vi "Default Position.vi"(0 "Selected Doc[]":refnum<class "Document.lvclass">[](array[class]), 5 "Position[]":T1[](array[typedef]), 11 "error in":errorcluster) -> (4 "Selected Doc[]":refnum<class "Document.lvclass">[](array[class]), 6 "Position[]":T1[](array[typedef]), 15 "error Out":errorcluster)   [LabVIEW 2016, in "LV MDI.lvclass"]
doc: "Set Default position for window."
uses:
  LV MDI.lvclass
  protected/Postion.ctl
  Document/Document base/Document.lvclass
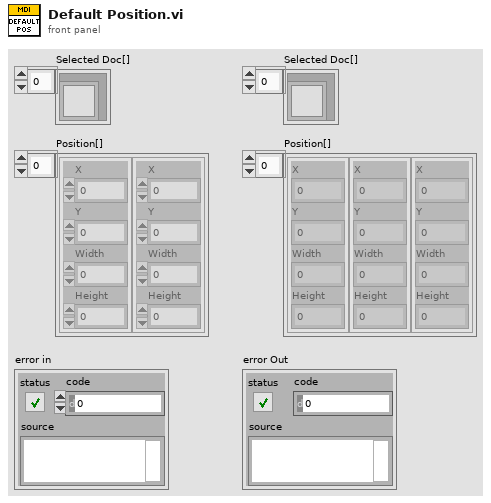
[diagram p1: front panel]
types:
  T1 = typedef "Postion.ctl" = cluster{"X":i32, "Y":i32, "Width":i32, "Height":i32}
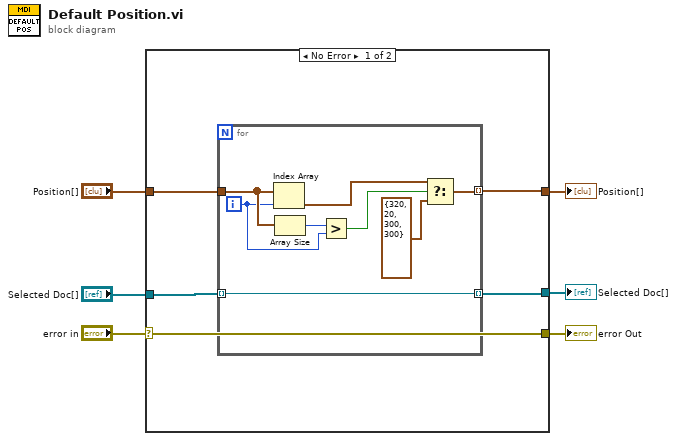
[diagram p0: block diagram]
diagram:
  n1 = case shown="No Error" "error in" {
    selector: "error in" -> [w7 w22]
    tunnel: [w10 w21] -> w6
    tunnel: "Position[]" -> [w9 w21]
    tunnel: "Selected Doc[]" -> [w8 w20]
    tunnel: [w7 w22] -> w2
    tunnel: [w11 w20] -> w1
    frame No Error {
      n2 = for {
        tunnel: w8 -> [w18] mode=indexing
        tunnel: w9 -> [w19]
        tunnel: [w14] -> w10 mode=indexing
        tunnel: [w18] -> w11 mode=indexing
        i -> [w16]
        n3 = Index Array(array=w19, index=w16) -> (element=w15:T1)
        n4 = Array Size(array=w19) -> (size(s)=w17:i32)
        n5 = Greater?(x=w17, y=w16) -> (0:w13:bool)
        n6 = Select(t=w15, s=w13, f=T1 {"X"=320, "Y"=20, "Width"=300, "Height"=300}) -> (s? t:f=w14:T1)
      }
    }
    frame Error {
    }
  }
  "Position[]" <- w6
  "error Out" <- w2
  "Selected Doc[]" <- w1
